vi "BeamProfile_SingleLineProc.vi"(8 "error in":errorcluster, 10 "initial parameters":dbl[](array[numeric])=[0.0, 1.0, 11.2, 0.02], 11 "data queue in":refnum<queue>) -> (0 "error out":errorcluster, 1 "Points/Fitted Curve":cluster{dbl[], dbl[]}[](array[cluster]), 2 "fit params":cluster{"z_pos":dbl, "fit_params":dbl[]}, 4 "R-square":dbl)   [LabVIEW 2013]
uses:
  <vilib>/Analysis/baseanly.llb/Mean (DBL).vi
  <vilib>/gmath/NumericalOptimization/Nonlinear Curve Fit LM.vi
  <vilib>/gmath/NI_Gmath.lvlib
  <vilib>/Analysis/NI_AALBase.lvlib
  <vilib>/Analysis/NI_AALPro.lvlib
panel:
  in  "Quit":bool
  out "raw+fit_profile":cluster{dbl[], "best nonlinear fit":dbl[]}[](graph)
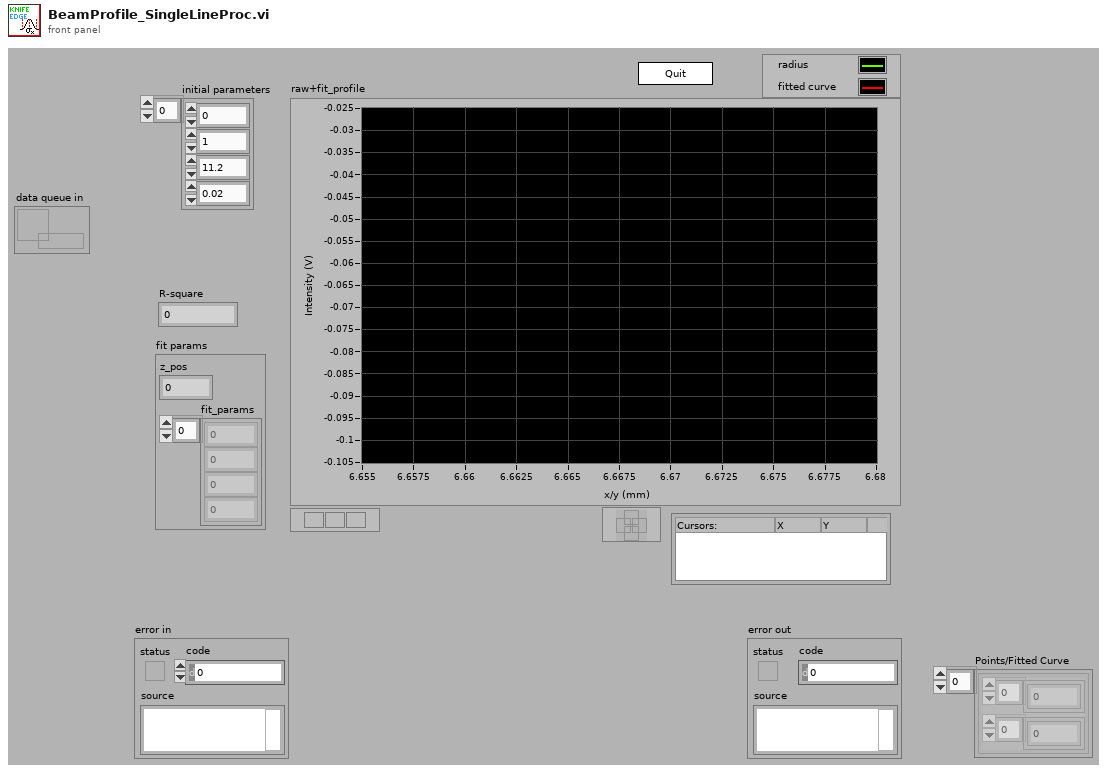
[diagram p1: front panel]
types:
  T1 = cluster{"X_micos":dbl, "Y_micos":dbl, "Spectra":sgl[]}
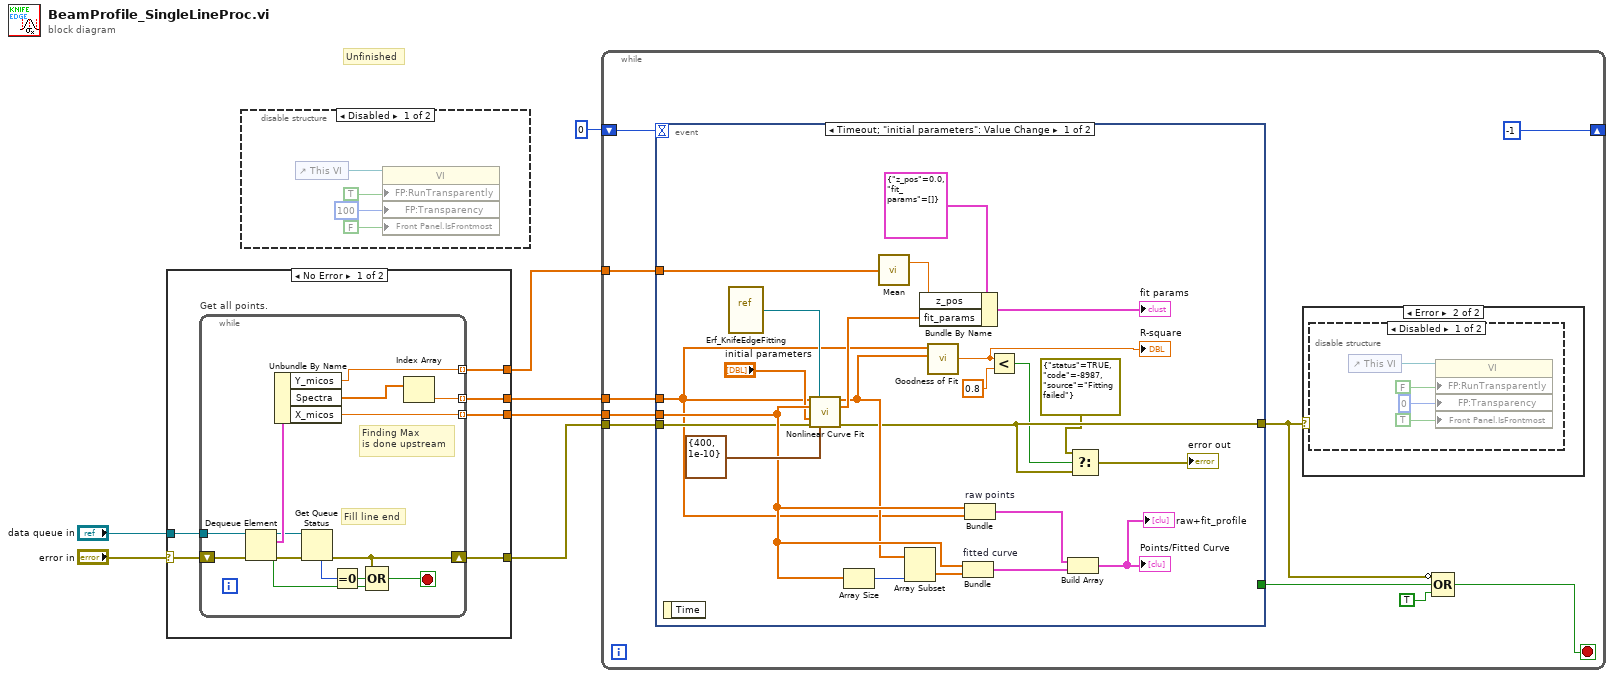
[diagram p0: block diagram]
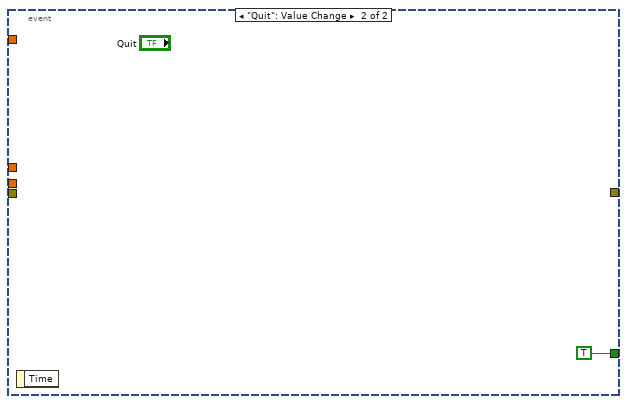
[diagram p5: hidden frame]
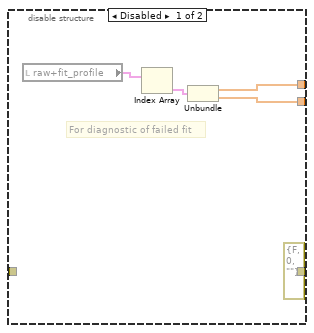
[diagram p7: hidden frame]
diagram:
  # "Unfinished"
  n1 = case shown="No Error" "error in" {
    selector: "error in" -> [w12 w27]
    tunnel: [w13 w28] -> w3
    tunnel: [w11 w30] -> w5
    tunnel: [w10 w29] -> w6
    tunnel: [w9 w29] -> w4
    tunnel: "data queue in" -> [w8 _]
    frame No Error {
      n2 = while "Get all points." {
        shift-right: [w18] -> w13
        shift-left: w12 -> [w26]
        tunnel: w8 -> [w25]
        tunnel: [w14] -> w11 mode=indexing
        tunnel: [w15] -> w10 mode=indexing
        tunnel: [w16] -> w9 mode=indexing
        stop <- w20 stop-if-true
        # "Finding Max\nis done upstream"
        # "Fill line end"
        n3 = Dequeue Element(queue=w25, error in (no error)=w26) -> (queue out=w23:refnum<queue>, element=w24:T1, timed out?=w19:bool, error out=w18:errorcluster)  [unwired: 1 in]
        n4 = Unbundle By Name(w24) -> ("Y_micos"=w16:dbl, "Spectra"=w17:sgl[], "X_micos"=w15:dbl)
        n5 = Get Queue Status(queue=w23) -> (# elements in queue=w22:i32)  [unwired: 2 in, 7 out]
        n6 = Equal To 0?(x=w22) -> (x = 0?=w21:bool)
        n7 = Compound Arithmetic op=OR(w18, w21, w19) -> (w20:bool)
        n8 = Index Array(array=w17) -> (element=w14:sgl)  [unwired: 1 in]
      }
    }
    frame Error {
      n9 = disable-structure shown="Enabled" {
        disable-tunnel: [w34 _] -> w30
        disable-tunnel: [w33 _] -> w29
        disable-tunnel: [errorcluster {"status"=FALSE, "code"=0, "source"=""} ("error IO") w36] -> w28
        disable-tunnel: w27 -> [_ w36]
        frame Disabled {
          # "For diagnostic of failed fit"
          n10 = local read "raw+fit_profile"() -> (w31:cluster{dbl[], "best nonlinear fit":dbl[]}[])
          n11 = Index Array(array=w31) -> (element=w35:cluster{dbl[], "best nonlinear fit":dbl[]})  [unwired: 1 in]
          n12 = Unbundle(w35) -> (w33:dbl[], "best nonlinear fit"=w34:dbl[])
        }
        frame Enabled {
        }
      }
    }
  }
  n13 = disable-structure shown="Disabled" {
    frame Disabled {
      n14 = control-ref of="This VI"() -> (w40:refnum<vi>)
      n15 = property class="VI"(reference=w40, "FP:RunTransparently"=TRUE ("Front Panel Window:Run VI Transparently"), "FP:Transparency"=u8 100 ("Front Panel Window:Transparency"), "Front Panel.IsFrontmost"=FALSE ("Front Panel Window:Is Frontmost")) -> ()  [unwired: 1 in, 2 out]
    }
    frame Enabled {
    }
  }
  n16 = while {
    tunnel: w6 -> [w50]
    tunnel: w5 -> [w49]
    tunnel: w4 -> [w48]
    tunnel: w3 -> [w47]
    shift-right: [-1] -> _
    shift-left: 0 -> [w46]
    stop <- w41 stop-if-true
    n17 = event shown="[0] Timeout;  \"initial parameters\": Value Change" {
      selector: _ -> [_ _]
      dyn-events: _ -> [_ _]
      timeout: w46 -> [_ _]
      tunnel: w50 -> [w73 _]
      tunnel: w49 -> [w61 _]
      tunnel: w48 -> [w72 _]
      tunnel: w47 -> [w67 _]
      tunnel: [w57 _] -> w43
      tunnel: [_ TRUE] -> w44
      event Timeout; "initial parameters": Value Change {
        n18 = event-data() -> ()  [unwired: 1 in, 1 out]
        n19 = vi-ref "Erf_KnifeEdgeFitting.vi"() -> (w76:refnum<vi>)
        n20 = call-poly <vilib>:"Nonlinear Curve Fit.vi"("Y"=w61, "f(x,a)"=w76, "X"=w73, "initial parameters"="initial parameters", "error in (no error)"=w67, "termination"=cluster{"max iteration":i32, "tolerance":dbl} {"max iteration"=400, "tolerance"=1e-10}) -> ("best nonlinear fit"=w62:dbl[], "best fit parameters"=w69:dbl[], "error out"=w57:errorcluster)  [unwired: 4 in, 3 out]
        n21 = Array Size(array=w73) -> (size(s)=w65:i32)
        n22 = call-poly <vilib>:"Mean.vi"("X"=w72) -> ("mean"=w77:dbl)  [unwired: 1 out]
        n23 = Array Subset(array=w62, length=w65) -> (w66:dbl[])  [unwired: 1 in]
        n24 = Bundle By Name(cluster=cluster{"z_pos":dbl, "fit_params":dbl[]} {"z_pos"=0.0, "fit_params"=[]}, "z_pos"=w77, "fit_params"=w69) -> (→"fit params":cluster{"z_pos":dbl, "fit_params":dbl[]})
        n25 = call <vilib>:"Goodness of Fit.vi"("Best Fit"=w62, "Y"=w61) -> ("R-square"=w59:dbl)  [unwired: 6 in, 3 out]
        "R-square" <- w59
        n26 = Bundle "fitted curve"(w73, w66) -> (w71:cluster{dbl[], dbl[]})  [unwired: 1 in]
        n27 = Bundle "raw points"(w73, "best nonlinear fit"=w61) -> (w70:cluster{dbl[], "best nonlinear fit":dbl[]})  [unwired: 1 in]
        n28 = Less?(x=w59, y=0.8) -> (x < y?=w55:bool)
        n29 = Build Array(w70, w71) -> (→"Points/Fitted Curve" →"raw+fit_profile":cluster{dbl[], "best nonlinear fit":dbl[]}[])
        n30 = Select(t=errorcluster {"status"=TRUE, "code"=-8987, "source"="Fitting failed"}, s=w55, f=w57) -> (s? t:f=→"error out":errorcluster)
      }
      event "Quit": Value Change {
        n31 = event-data() -> ()  [unwired: 1 in, 1 out]
      }
    }
    n32 = case shown="Error" w43 {
      frame No Error {
      }
      frame Error {
        n33 = disable-structure shown="Disabled" {
          frame Disabled {
            n34 = control-ref of="This VI"() -> (w51:refnum<vi>)
            n35 = property class="VI"(reference=w51, "FP:RunTransparently"=FALSE ("Front Panel Window:Run VI Transparently"), "FP:Transparency"=u8 0 ("Front Panel Window:Transparency"), "Front Panel.IsFrontmost"=TRUE ("Front Panel Window:Is Frontmost")) -> ()  [unwired: 1 in, 2 out]
          }
          frame Enabled {
          }
        }
      }
    }
    n36 = Compound Arithmetic op=OR(invert w43, w44, TRUE) -> (w41:bool)
  }
